vi "Initialize Photodiodes.vi"() -> (0 "error out":errorcluster, 1 "Sample Rate (Hz)":dbl=1000000.0 format="%0.2f", 2 "Time to sample (seconds)":dbl=2.0, 3 "task out":refnum<k21>)   [LabVIEW 2018]
uses:
  <vilib>/DAQmx/create/channels.llb/DAQmx Create Channel (AI-Voltage-Basic).vi
  <vilib>/DAQmx/configure/timing.llb/DAQmx Timing (Sample Clock).vi
  <vilib>/DAQmx/configure/trigger.llb/DAQmx Start Trigger (None).vi
panel:
  in  "Buffer size (samples per channel)":u32=2000384
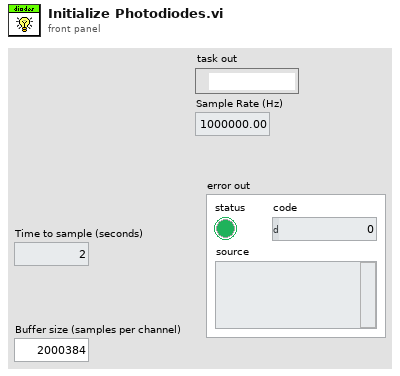
[diagram p1: front panel]
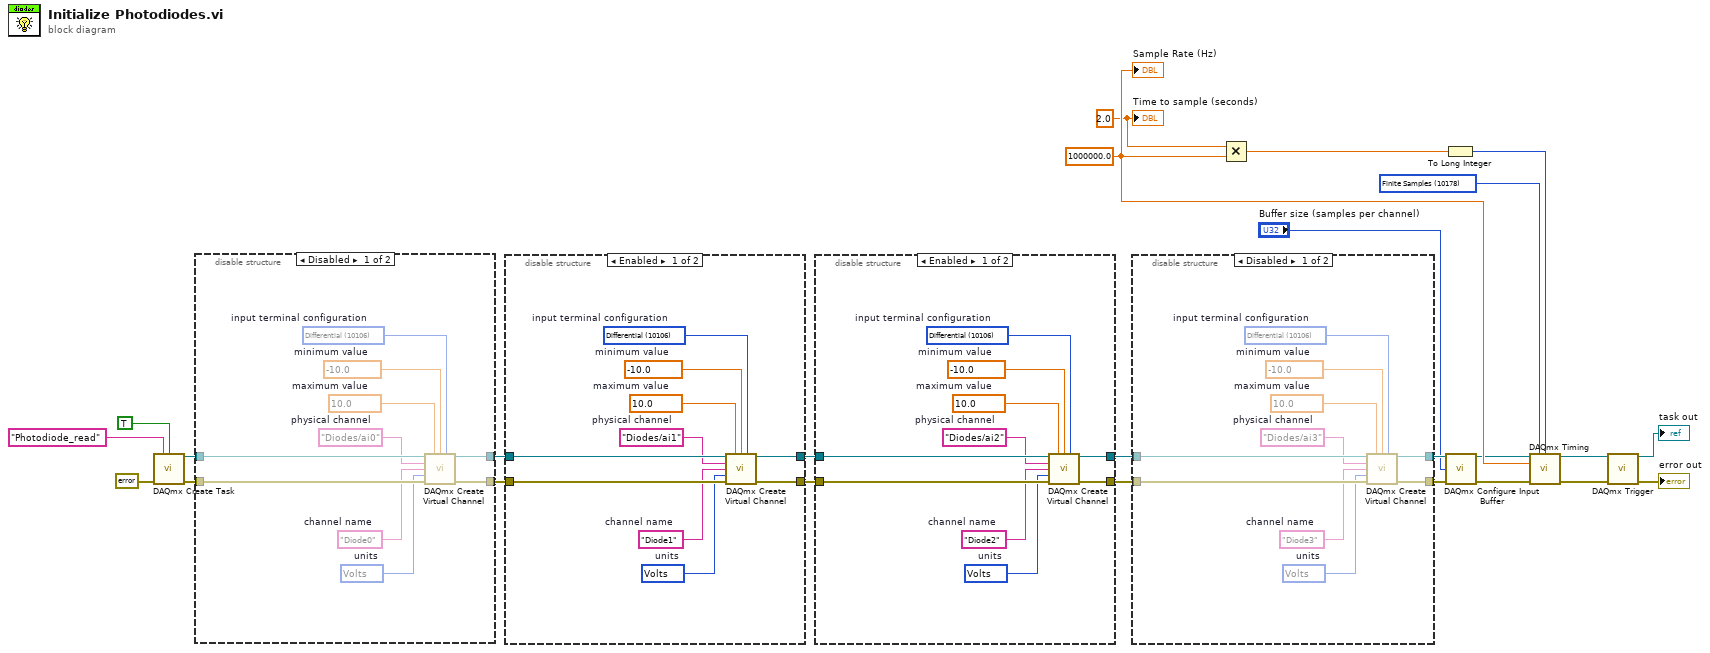
[diagram p0: block diagram]
diagram:
  w17 = 1000000.0 ("Sample Rate (Hz)")
  w1 = 2.0 ("Time to sample (seconds)")
  w21 = 10178 items=["Finite Samples"=10178, "Continuous Samples"=10123, "Hardware Timed Single Point"=12522] ("sample mode")
  n1 = call <vilib>:"DAQmx Create Task.vi"("new task name"="Photodiode_read", "auto cleanup"=TRUE, "error in"=errorcluster {"status"=FALSE, "code"=0, "source"=""}) -> ("task out"=w23:refnum<k21>, "error out"=w25:errorcluster)  [unwired: 11 in]
  n2 = disable-structure shown="Disabled" {
    disable-tunnel: w25 -> [w35 w36]
    disable-tunnel: w23 -> [w34 w37]
    disable-tunnel: [w30 w36] -> w20
    disable-tunnel: [w26 w37] -> w19
    frame Disabled {
      w27 = 10106 items=["default"=-1, "RSE"=10083, "NRSE"=10078, "Differential"=10106, "Pseudodifferential"=12529]  # input terminal configuration
      w28 = 10348 items=["Volts"=10348, "From Custom Scale"=10065]  # units
      w29 = "Diode0"  # channel name
      w31 = -10.0  # minimum value
      w32 = 10.0  # maximum value
      w33 = "Diodes/ai0"  # physical channel
      n3 = call-poly <vilib>:"DAQmx Create Virtual Channel.vi"("task in"=w34, "maximum value"=w32, "minimum value"=w31, "input terminal configuration"=w27, "physical channels"=w33, "name to assign"=w29, "units"=w28, "error in"=w35) -> ("task out"=w26:refnum<k21>, "error out"=w30:errorcluster)  [unwired: 6 in]
    }
    frame Enabled {
    }
  }
  n4 = disable-structure shown="Enabled" {
    disable-tunnel: w20 -> [w47 w48]
    disable-tunnel: w19 -> [w46 w49]
    disable-tunnel: [w42 w48] -> w15
    disable-tunnel: [w38 w49] -> w14
    frame Enabled {
      w39 = 10106 items=["default"=-1, "RSE"=10083, "NRSE"=10078, "Differential"=10106, "Pseudodifferential"=12529]  # input terminal configuration
      w40 = 10348 items=["Volts"=10348, "From Custom Scale"=10065]  # units
      w41 = "Diode1"  # channel name
      w43 = -10.0  # minimum value
      w44 = 10.0  # maximum value
      w45 = "Diodes/ai1"  # physical channel
      n5 = call-poly <vilib>:"DAQmx Create Virtual Channel.vi"("task in"=w46, "maximum value"=w44, "minimum value"=w43, "input terminal configuration"=w39, "physical channels"=w45, "name to assign"=w41, "units"=w40, "error in"=w47) -> ("task out"=w38:refnum<k21>, "error out"=w42:errorcluster)  [unwired: 6 in]
    }
    frame Disabled {
    }
  }
  n6 = disable-structure shown="Enabled" {
    disable-tunnel: w15 -> [w59 w61]
    disable-tunnel: w14 -> [w58 w60]
    disable-tunnel: [w57 w61] -> w13
    disable-tunnel: [w56 w60] -> w12
    frame Enabled {
      w50 = 10106 items=["default"=-1, "RSE"=10083, "NRSE"=10078, "Differential"=10106, "Pseudodifferential"=12529]  # input terminal configuration
      w51 = 10348 items=["Volts"=10348, "From Custom Scale"=10065]  # units
      w52 = "Diode2"  # channel name
      w53 = -10.0  # minimum value
      w54 = 10.0  # maximum value
      w55 = "Diodes/ai2"  # physical channel
      n7 = call-poly <vilib>:"DAQmx Create Virtual Channel.vi"("task in"=w58, "maximum value"=w54, "minimum value"=w53, "input terminal configuration"=w50, "physical channels"=w55, "name to assign"=w52, "units"=w51, "error in"=w59) -> ("task out"=w56:refnum<k21>, "error out"=w57:errorcluster)  [unwired: 6 in]
    }
    frame Disabled {
    }
  }
  n8 = disable-structure shown="Disabled" {
    disable-tunnel: [w71 w72] -> w7
    disable-tunnel: [w70 w73] -> w10
    disable-tunnel: w13 -> [w69 w73]
    disable-tunnel: w12 -> [w68 w72]
    frame Disabled {
      w63 = 10106 items=["default"=-1, "RSE"=10083, "NRSE"=10078, "Differential"=10106, "Pseudodifferential"=12529]  # input terminal configuration
      w64 = 10348 items=["Volts"=10348, "From Custom Scale"=10065]  # units
      w62 = "Diode3"  # channel name
      w65 = -10.0  # minimum value
      w66 = 10.0  # maximum value
      w67 = "Diodes/ai3"  # physical channel
      n9 = call-poly <vilib>:"DAQmx Create Virtual Channel.vi"("task in"=w68, "maximum value"=w66, "minimum value"=w65, "input terminal configuration"=w63, "physical channels"=w67, "name to assign"=w62, "units"=w64, "error in"=w69) -> ("task out"=w71:refnum<k21>, "error out"=w70:errorcluster)  [unwired: 6 in]
    }
    frame Enabled {
    }
  }
  n10 = Multiply(x=w1, y=w17) -> (x*y=w16:dbl)
  n11 = To Long Integer(number=w16) -> (32bit integer=w11:i32)
  n12 = call <vilib>:"DAQmx Configure Input Buffer.vi"("task/channels in"=w7, "buffer size (in samples per channel)"="Buffer size (samples per channel)", "error in"=w10) -> ("task out"=w8:refnum<k21>, "error out"=w9:errorcluster)  [unwired: 11 in]
  n13 = call-poly <vilib>:"DAQmx Timing.vi"("task/channels in"=w8, "sample mode"=w21, "samples per channel"=w11, "rate"=w17, "error in"=w9) -> ("task out"=w3:refnum<k21>, "error out"=w5:errorcluster)  [unwired: 9 in]
  n14 = call-poly <vilib>:"DAQmx Trigger.vi"("task/channels in"=w3, "error in"=w5) -> ("task out"=→"task out":refnum<k21>, "error out"=→"error out":errorcluster)  [unwired: 12 in]
  "Time to sample (seconds)" <- w1
  "Sample Rate (Hz)" <- w17
